vi "Read-Write Debug Status.vi"(4 "error in (no error)":errorcluster, 5 "Debug Tag (\"\")":string, 6 "Debugged VI Name (\"\")":string, 7 "Debug Ref":T1) -> (0 "error out":errorcluster, 2 "DEBUG?":bool, 3 "dup Debug Ref":T1)   [LabVIEW 2011]
uses:
  <vilib>/Utility/config.llb/Config Data RefNum.ctl
  <vilib>/Utility/config.llb/Read Key (Boolean).vi
  <vilib>/Utility/config.llb/Write Key (Boolean).vi
  <vilib>/Utility/config.llb/NI_LVConfig.lvlib
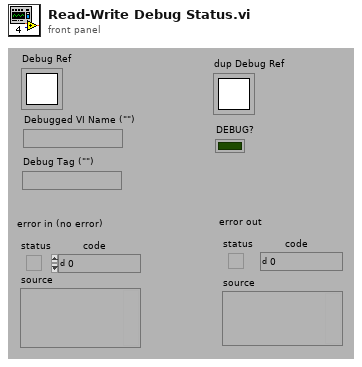
[diagram p1: front panel]
types:
  T1 = typedef "NI_LVConfig.lvlib/Config Data RefNum.ctl" = refnum<k1>
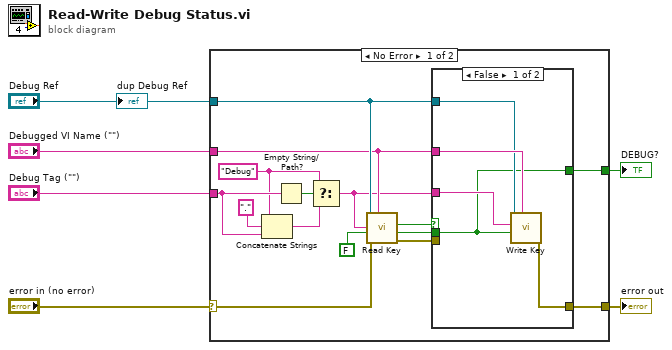
[diagram p0: block diagram]
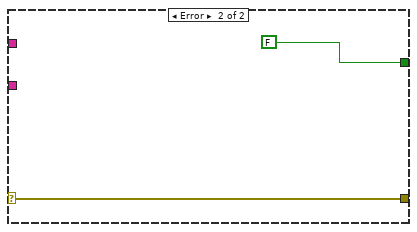
[diagram p3: hidden frame]
diagram:
  n1 = case shown="No Error" "error in (no error)" {
    selector: "error in (no error)" -> [w15 w29]
    tunnel: [w13 FALSE] -> w5
    tunnel: [w12 w29] -> w4
    tunnel: "Debugged VI Name (\"\")" -> [w11 _]
    tunnel: "Debug Ref" -> [w14 _]
    tunnel: "Debug Tag (\"\")" -> [w21 _]
    frame No Error {
      w18 = "Debug"
      n2 = Concatenate Strings(w18, ".", w21) -> (w17:string)
      n3 = Empty String/Path?(string/path=w21) -> (empty?=w19:bool)
      n4 = Select(t=w18, s=w19, f=w17) -> (s? t:f=w7:string)
      n5 = call-poly <vilib>:"Read Key.vi"("section"=w11, "error in (no error)"=w15, "default value"=FALSE, "key"=w7, "refnum"=w14) -> ("error out"=w8:errorcluster, "value"=w10:bool, "found?"=w9:bool)  [unwired: 4 out]
      n6 = case shown="False" w9 {
        tunnel: w14 -> [w25 _]
        tunnel: [w22 w28] -> w13
        tunnel: w10 -> [w22 w28]
        tunnel: [w24 w27] -> w12
        tunnel: w11 -> [w26 _]
        tunnel: w8 -> [_ w27]
        tunnel: w7 -> [w23 _]
        frame False {
          n7 = call-poly <vilib>:"Write Key.vi"("section"=w26, "value"=w22, "key"=w23, "refnum"=w25) -> ("error out"=w24:errorcluster)  [unwired: 1 in, 6 out]
        }
        frame True {
        }
      }
    }
    frame Error {
    }
  }
  "error out" <- w4
  "DEBUG?" <- w5
  "dup Debug Ref" <- "Debug Ref"
